vi "main_NI-IMAQ.vi"   [LabVIEW 2013]
types:
  T1 = typedef "Image Type" = u32
  T2 = typedef "IMAQ Image.ctl" = refnum<image>
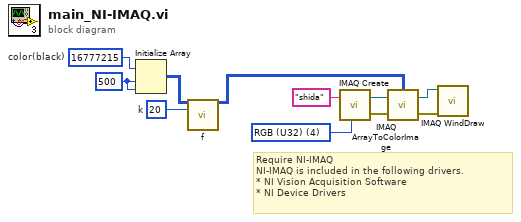
[diagram p0: block diagram]
diagram:
  w7 = T1 4 items=["Grayscale (U8)", "Grayscale (I16)", "Grayscale (SGL)", "Complex (CSG)", "RGB (U32)", "HSL (U32)", "RGB (U64)", "Grayscale (U16)"] ("Image Type")
  w8 = u32 16777215  # color(black)
  w10 = 500 ("次元サイズ")
  w11 = 20  # k
  # "Require NI-IMAQ\nNI-IMAQ is included in the following drivers.\n* NI Vision Acquisition Software\n* NI Device Drivers"
  n1 = Initialize Array(w8, w10, w10) -> (w9:u32[][])
  n2 = call "f.vi"("配列"=w9, "k"=w11) -> ("配列 2"=w6:u32[][])  [unwired: 12 in, 1 out]
  n3 = call "IMAQ Create"("Image Name"="shida", "Image Type"=w7) -> ("New Image"=w4:T2, "error out"=w3:errorcluster)  [unwired: 3 in]
  n4 = call "IMAQ ArrayToColorImage"("Image Pixels (U32)"=w6, "Image"=w4, "error in (no error)"=w3) -> ("Image Out"=w2:T2, "error out"=w1:errorcluster)  [unwired: 2 in]
  n5 = call "IMAQ WindDraw"("error in (no error)"=w1, "Image"=w2) -> ()  [unwired: 8 in, 2 out]
